vi "Param_setup.vi"(1 "Offset":dbl format="%#_13g", 2 "Phase Marker (deg)":dbl format="%#_13g", 3 "Trig Link Line":i32, 4 "Frequency":dbl format="%#_13g", 5 "Phase Marker?":bool=TRUE, 6 "Amplitude":dbl format="%#_13g") -> (0 "Sine Wave Params 2":T1={"Frequency (Hz)"=1000.0, "Amplitude (A)"=0.001, "Offset (A)"=0.0, "Ranging Mode"=enum."Best", "Fixed Range"=enum."2mA", "Playback Mode"=enum."Time", "Time (s)"=1.0, "Num Cycles"=1.0, "Phase\nMarker?"=FALSE, "Phase Marker (deg)"=180.0, "Trig Link Line"=enum."1"} {"Offset (A)" min=-0.105 max=0.105 format="%.4p"; "Num Cycles" min=0.001 max=99999999900.0 format="%.3p"; "Time (s)" min=1e-07 max=999999.999 format="%.3p"; "Phase Marker (deg)" min=0.0 max=360.0 format="%.3f"; "Amplitude (A)" min=2e-12 max=0.105 format="%.3p"; "Frequency (Hz)" min=0.001 max=100000.0 format="%.3p"})   [LabVIEW 2014]
uses:
  Equipment/Keithley 6221/Configure/6221 Wave/Typedefs/KE6221 -- Wave Sine Wave Params.ctl
  Equipment/Keithley 6221/Configure/6221 Wave/Low Level/Typedefs/KE6221 -- Wave Frequency.ctl
  Equipment/Keithley 6221/Configure/6221 Wave/Low Level/Typedefs/KE6221 -- Wave Amplitude.ctl
  Equipment/Keithley 6221/Configure/Source/Typedefs/KE622x -- Current Level.ctl
  Equipment/Keithley 6221/Configure/6221 Wave/Low Level/Typedefs/KE6221 -- Wave Ranging Mode.ctl
  Equipment/Keithley 6221/Configure/Source/Typedefs/KE622x -- Current Ranges.ctl
  Equipment/Keithley 6221/Configure/6221 Wave/Low Level/Typedefs/KE6221 -- Wave Playback Mode.ctl
  Equipment/Keithley 6221/Configure/6221 Wave/Low Level/Typedefs/KE6221 -- Wave Playback Time.ctl
  Equipment/Keithley 6221/Configure/6221 Wave/Low Level/Typedefs/KE6221 -- Wave Playback Num Cycles.ctl
  Equipment/Keithley 6221/Configure/6221 Wave/Low Level/Typedefs/KE6221 -- Wave Phase Marker.ctl
  Equipment/Keithley 6221/Configure/Trigger/Low Level/Typedefs/KE622x -- Trig Link Line.ctl
  Equipment/Keithley 6221/Keithley 622x.lvlib
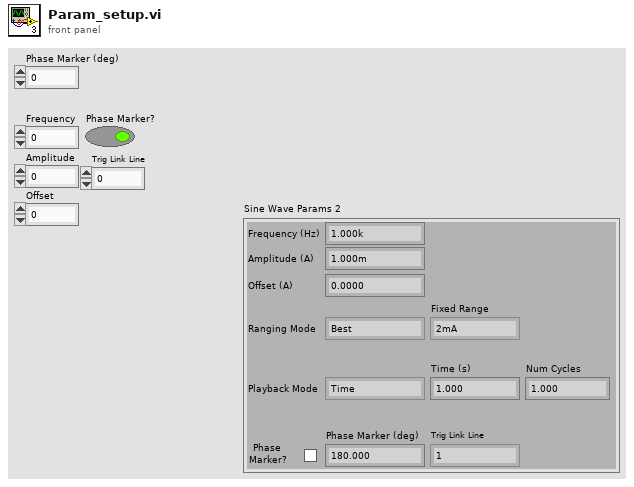
[diagram p1: front panel]
types:
  T1 = typedef "Keithley 622x.lvlib/KE6221 -- Wave Sine Wave Params.ctl" = cluster{"Frequency (Hz)":T2, "Amplitude (A)":T3, "Offset (A)":T4, "Ranging Mode":T5, "Fixed Range":T6, "Playback Mode":T7, "Time (s)":T8, "Num Cycles":T9, "Phase\nMarker?":bool, "Phase Marker (deg)":T10, "Trig Link Line":T11}
  T2 = typedef "Keithley 622x.lvlib/KE6221 -- Wave Frequency.ctl" = dbl
  T3 = typedef "Keithley 622x.lvlib/KE6221 -- Wave Amplitude.ctl" = dbl
  T4 = typedef "Keithley 622x.lvlib/KE622x -- Current Level.ctl" = dbl
  T5 = typedef "Keithley 622x.lvlib/KE6221 -- Wave Ranging Mode.ctl" = enum16{"Best", "Fixed"}
  T6 = typedef "Keithley 622x.lvlib/KE622x -- Current Ranges.ctl" = enum16{"2nA", "20nA", "200nA", "2uA", "20uA", "200uA", "2mA", "20mA", "100mA"}
  T7 = typedef "Keithley 622x.lvlib/KE6221 -- Wave Playback Mode.ctl" = enum16{"Time", "Num Cycles"}
  T8 = typedef "Keithley 622x.lvlib/KE6221 -- Wave Playback Time.ctl" = dbl
  T9 = typedef "Keithley 622x.lvlib/KE6221 -- Wave Playback Num Cycles.ctl" = dbl
  T10 = typedef "Keithley 622x.lvlib/KE6221 -- Wave Phase Marker.ctl" = dbl
  T11 = typedef "Keithley 622x.lvlib/KE622x -- Trig Link Line.ctl" = enum16{"1", "2", "3", "4", "5", "6"}
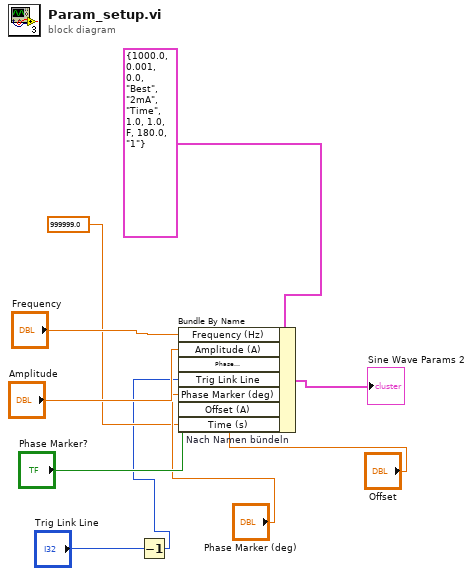
[diagram p0: block diagram]
diagram:
  n1 = Decrement(x="Trig Link Line") -> (x-1=w2:i32)
  n2 = Bundle By Name "Nach Namen bündeln"(cluster=T1 {"Frequency (Hz)"=1000.0, "Amplitude (A)"=0.001, "Offset (A)"=0.0, "Ranging Mode"=enum."Best", "Fixed Range"=enum."2mA", "Playback Mode"=enum."Time", "Time (s)"=1.0, "Num Cycles"=1.0, "Phase\nMarker?"=FALSE, "Phase Marker (deg)"=180.0, "Trig Link Line"=enum."1"} ("Sine Wave Params"), "Frequency (Hz)"="Frequency", "Amplitude (A)"="Amplitude", "Phase\nMarker?"="Phase Marker?", "Trig Link Line"=w2, "Phase Marker (deg)"="Phase Marker (deg)", "Offset (A)"="Offset", "Time (s)"=999999.0) -> (→"Sine Wave Params 2":T1)
